vi "Configure Data Buffer.vi"(0 "VISA resource name":refnum<visa-resource-name>, 5 "buffer (1:Buffer 1)":u16(ring)=1 items=["Buffer 1"=1, "Buffer 2"=2], 7 "Enable buffer feed (T)":bool=TRUE, 9 "function (1:primary)":u16(ring)=1 items=["primary"=1, "secondary"=2], 11 "error in (no error)":errorcluster, 12 "number of points (10)":i16=10 min=1 max=200 step=1) -> (4 "VISA resource name out":refnum<visa-resource-name>, 15 "error out":errorcluster)   [LabVIEW 2016, in "Agilent 4263X.lvlib"]
doc: "This VI configures the data buffer(s) of the instrument. \n\nThis VI should be executed before the Read Data Buffer VI is used."
uses:
  <instrlib>/Agilent 4263X/Agilent 4263X.lvlib
panel:
  # "yes\nno"
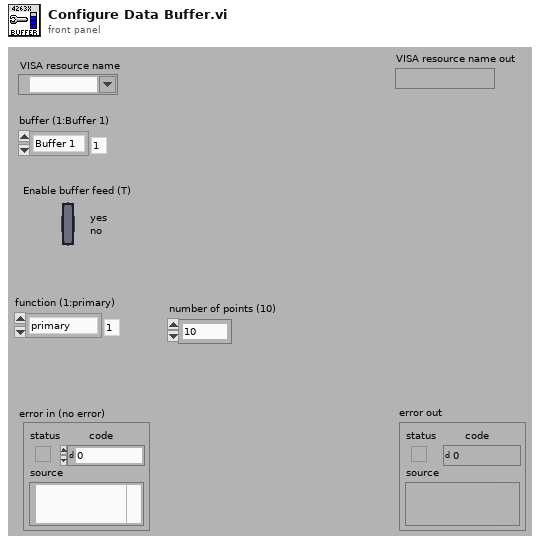
[diagram p1: front panel]
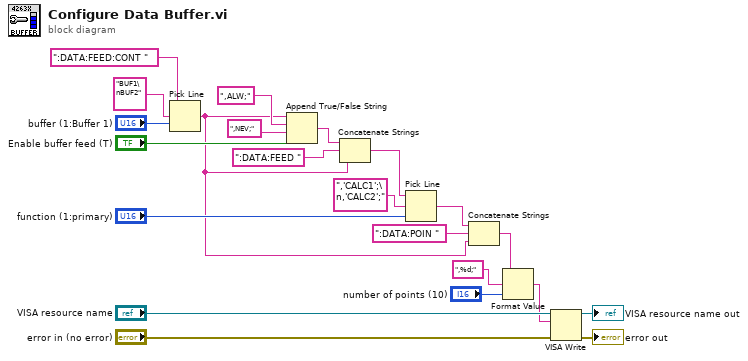
[diagram p0: block diagram]
diagram:
  n1 = Pick Line(string ("")=":DATA:FEED:CONT ", multi-line string="BUF1\nBUF2", line index="buffer (1:Buffer 1)") -> (output string=w1:string)
  n2 = Append True/False String(1:"Enable buffer feed (T)", 2:",NEV;", 3:",ALW;", 4:w1) -> (0:w9:string)
  n3 = Concatenate Strings(w9, ":DATA:FEED ", w1) -> (w4:string)
  n4 = Pick Line(string ("")=w4, multi-line string=",'CALC1';\n,'CALC2';", line index="function (1:primary)") -> (output string=w8:string)
  n5 = Concatenate Strings(w8, ":DATA:POIN ", w1) -> (w12:string)
  n6 = Format Value(string ("")=w12, format string=",%d;", value (0)="number of points (10)") -> (output string=w7:string)
  n7 = VISA Write(VISA resource name="VISA resource name", write buffer=w7, error in (no error)="error in (no error)") -> (VISA resource name out=→"VISA resource name out":refnum<visa-resource-name>, error out=→"error out":errorcluster)  [unwired: 1 out]
